vi "API_DB.GetAllMaterials.vi"(0 "Database in":refnum<class "Database.lvclass">, 1 "Wait (F)":bool, 11 "error in (no error)":errorcluster, 12 "Timeout (ms)":u32) -> (4 "Database out":refnum<class "Database.lvclass">, 6 "Materials":string[](array[string]), 15 "error out":errorcluster)   [LabVIEW 2022 SP3, in "Database.lvclass"]
doc: "Developed by Kevin Thompson\nkevin@thompsonengineering.net\n\nCopyright 2018\nThompson Engineering, LLC"
uses:
  Database.lvclass
  DataTypes/AsynCmd_Temp01--enum.ctl
  DataTypes/QuiryBuilderData--Cluster.ctl
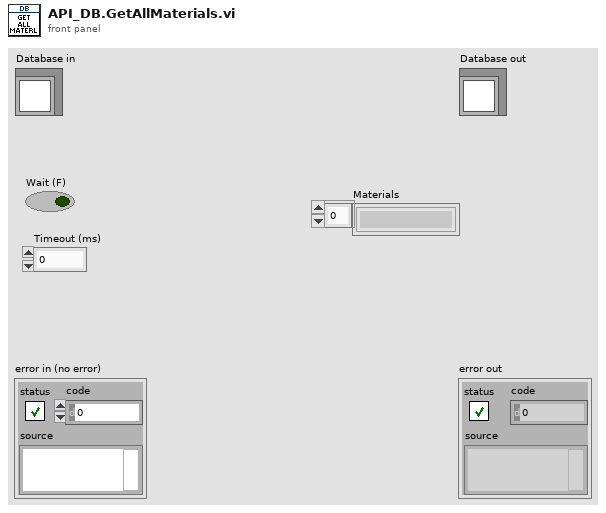
[diagram p1: front panel]
types:
  T1 = typedef "QuiryBuilderData--Cluster.ctl" = cluster{"Table":string, "Column":string[], "Value":string[], "WhereColumn":string[], "WhereValue":string[], "OrderBy":string[]}
  T2 = typedef "Database.lvclass/AsynCmd_Temp01--enum.ctl" = enum16{"DB.DeleteRecord", "DB.UpdateRecord", "DB.InsertRecord", "DB.SelectRecord", "DB.ExecuteSQLCommand", "DB.FindFirstSlot", "DB.GenericSQLQuery"}
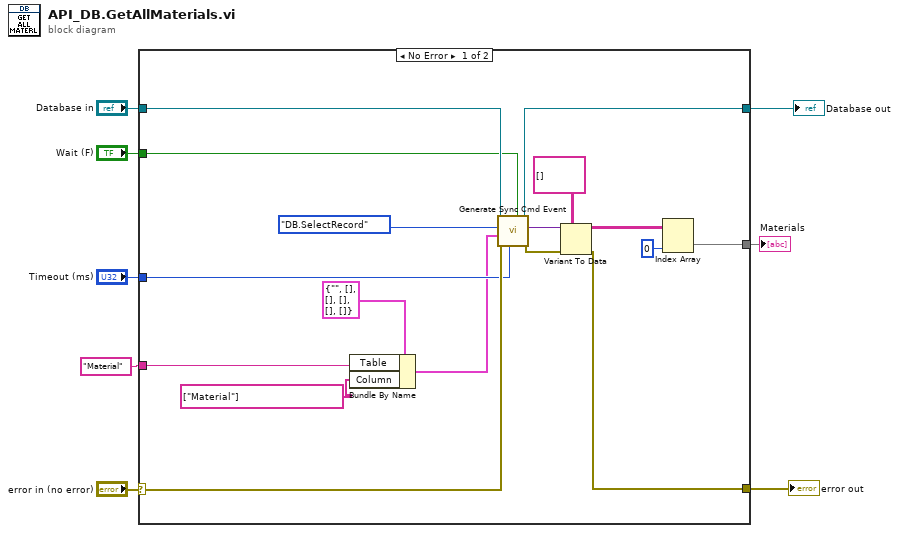
[diagram p0: block diagram]
diagram:
  n1 = case shown="No Error" "error in (no error)" {
    selector: "error in (no error)" -> [w23 w27]
    tunnel: [w19 w27] -> w7
    tunnel: [w24 w26] -> w5
    tunnel: "Database in" -> [w25 w26]
    tunnel: "Wait (F)" -> [w18 _]
    tunnel: "Timeout (ms)" -> [w17 _]
    tunnel: "Material" ("Table") -> [w15 _]
    tunnel: [w9 _] -> w1
    frame No Error {
      n2 = Bundle By Name(cluster=T1 {"Table"="", "Column"=[], "Value"=[], "WhereColumn"=[], "WhereValue"=[], "OrderBy"=[]} ("QueryBuilderData"), "Table"=w15, "Column"=string[] ["Material"]) -> (w16:T1)
      n3 = call "Generate Sync Cmd Event.vi"("Wait (F)"=w18, "Timeout (ms)"=w17, "error in (no error)"=w23, "vData"=w16, "AsyncCmd"=AsynCmd_Temp01--enum."DB.SelectRecord", "Database in"=w25) -> ("error out"=w20:errorcluster, "Return Value"=w21:variant, "Database out"=w24:refnum<class "Database.lvclass">)  [unwired: 3 in]
      n4 = Variant To Data(error in=w20, type=string[][] [], Variant=w21) -> (data=w11:string[][], error out=w19:errorcluster)
      n5 = Index Array(array=w11, index (col)=0 ("disabled index (col)")) -> (element=w9:string[])  [unwired: 1 in]
    }
    frame Error {
    }
  }
  "error out" <- w7
  "Database out" <- w5
  "Materials" <- w1
